vi "support.vi"() -> ()   [LabVIEW 2017]
panel:
  out "appended array":dbl[][](array[numeric])
  out "tf (s)":dbl
  in  "Velocity (mm/s)":dbl=100.0
  in  "Target":cluster{"Xf":dbl, "Yf":dbl}
  in  "Start Point":cluster{"X0":dbl, "Y0":dbl}
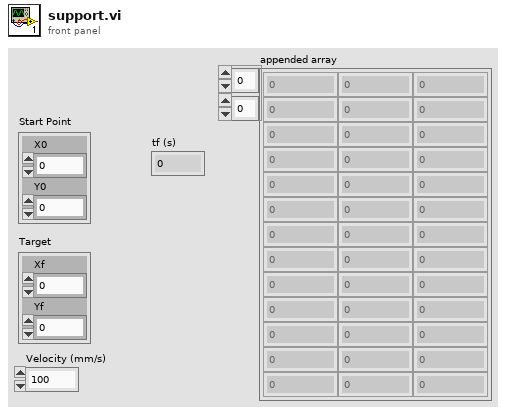
[diagram p1: front panel]
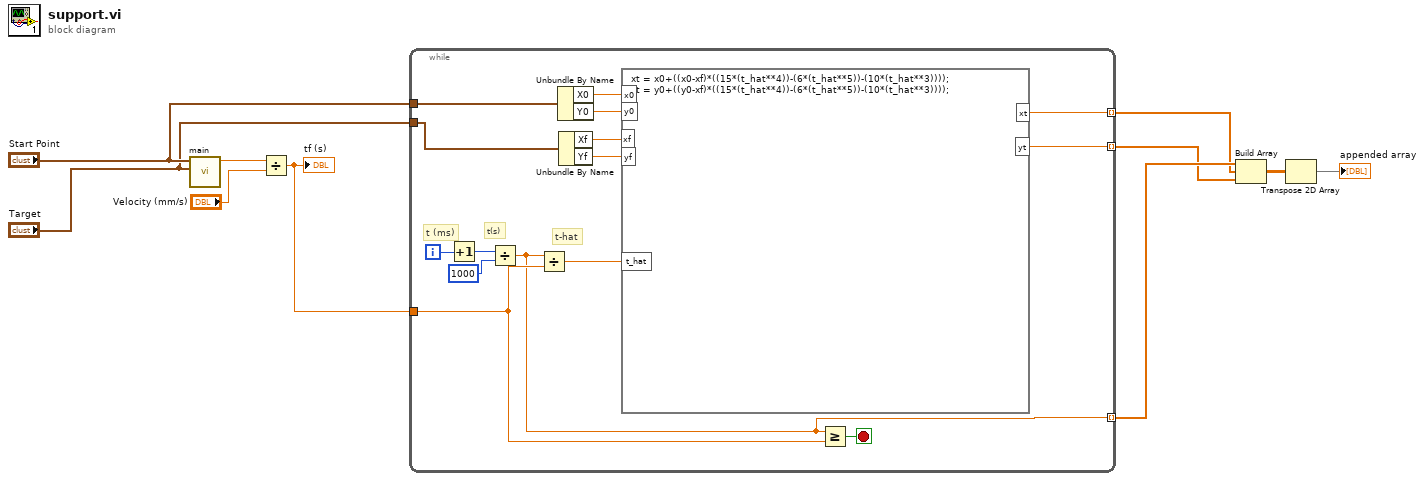
[diagram p0: block diagram]
diagram:
  n1 = call "main.vi"("Target"="Target", "Start Point"="Start Point") -> ("Distance (mm)"=w10:dbl)  [unwired: 9 in]
  n2 = Divide(x=w10, y="Velocity (mm/s)") -> (x/y=w6:dbl)
  "tf (s)" <- w6
  n3 = while {
    tunnel: "Start Point" -> [w19]
    tunnel: "Target" -> [w16]
    tunnel: w6 -> [w22]
    tunnel: [w13] -> w4 mode=indexing
    tunnel: [w12] -> w3 mode=indexing
    tunnel: [w11] -> w5 mode=indexing
    i -> [w25]
    stop <- w21 stop-if-true
    # "t-hat"
    # "t(s)"
    # "t (ms)"
    n4 = Increment(x=w25) -> (x+1=w24:i32)
    n5 = Divide(x=w24, y=1000) -> (x/y=w11:dbl)
    n6 = Divide(x=w11, y=w22) -> (x/y=w20:dbl)
    n7 = Unbundle By Name(w19) -> ("X0"=w18:dbl, "Y0"=w17:dbl)
    n8 = Unbundle By Name(w16) -> ("Xf"=w15:dbl, "Yf"=w14:dbl)
    n9 = formula code="xt = x0+((x0-xf)*((15*(t_hat**4))-(6*(t_hat**5))-(10*(t_hat**3))));\nyt = y0+((y0-xf)*((15*(t_hat**4))-(6*(t_hat**5))-(10*(t_hat**3))));"("t_hat"=w20, "x0"=w18, "y0"=w17, "xf"=w15, "yf"=w14) -> ("xt"=w13:dbl, "yt"=w12:dbl)
    n10 = Greater Or Equal?(x=w11, y=w22) -> (x >= y?=w21:bool)
  }
  n11 = Build Array(w5, w4, w3) -> (w2:dbl[][])
  n12 = Transpose 2D Array(2D array=w2) -> (transposed array=→"appended array":dbl[][])
